vi "controller.vi"() -> ()   [LabVIEW 2017]
uses:
  <vilib>/Instr/_visa.llb/VISA Configure Serial Port (Instr).vi
panel:
  in  "7":bool
  in  "9":bool
  in  "8":bool
  in  "5":bool
  in  "6":bool
  in  "4":bool
  in  "3":bool
  in  "2":bool
  in  "1":bool
  in  "5-3":bool
  in  "5-1":bool
  in  "10-3":bool
  in  "10-2":bool
  in  "10-1":bool
  in  "9-5":bool
  in  "9-4":bool
  in  "9-3":bool
  in  "9-2":bool
  in  "9-1":bool
  in  "8-5":bool
  in  "8-4":bool
  in  "8-3":bool
  in  "8-2":bool
  in  "8-1":bool
  in  "7-5":bool
  in  "7-4":bool
  in  "7-3":bool
  in  "7-2":bool
  in  "7-1":bool
  in  "6-5":bool
  in  "6-4":bool
  in  "6-3":bool
  in  "6-2":bool
  in  "6-1":bool
  in  "5-5":bool
  in  "5-4":bool
  in  "5-2":bool
  in  "4-5":bool
  in  "4-4":bool
  in  "4-3":bool
  in  "4-2":bool
  in  "4-1":bool
  in  "3-5":bool
  in  "3-4":bool
  in  "3-3":bool
  in  "3-2":bool
  in  "3-1":bool
  in  "2-5":bool
  in  "2-4":bool
  in  "2-3":bool
  in  "2-2":bool
  in  "2-1":bool
  in  "1-5":bool
  in  "1-4":bool
  in  "1-3":bool
  in  "1-2":bool
  in  "1-1":bool
  in  "关":u16(ring) items=["1", "2", "3", "4", "5", "6", "7", "8", "9", "10", "11", "12", "13", "14", "15", "16", "17", "18", "19", "20", "21", "22", "23", "24", "25", "26", "27", "28", "29", "30", "31", "32", "33", "34", "35", "36", "37", "38", "39", "40", "41", "42", "43", "44", "45", "46", "47", "48"]
  in  "开":u16(ring) items=["1", "2", "3", "4", "5", "6", "7", "8", "9", "10", "11", "12", "13", "14", "15", "16", "17", "18", "19", "20", "21", "22", "23", "24", "25", "26", "27", "28", "29", "30", "31", "32", "33", "34", "35", "36", "37", "38", "39", "40", "41", "42", "43", "44", "45", "46", "47", "48"]
  in  "全关":bool
  in  "全开":bool
  in  "控制板":refnum<visa-resource-name>="COM9"
  in  "退出":bool
  in  "传感器预热完成":bool
  in  "传感器预热":bool
  in  "流程测试":bool
  in  "测试":bool
  in  "传感器数目":i32=9
  # "控制板调试"
  # "注意：\n因串口带宽、通信时延与寄存器读写操作，\n点击按钮后请等待反应。不要反复点击。"
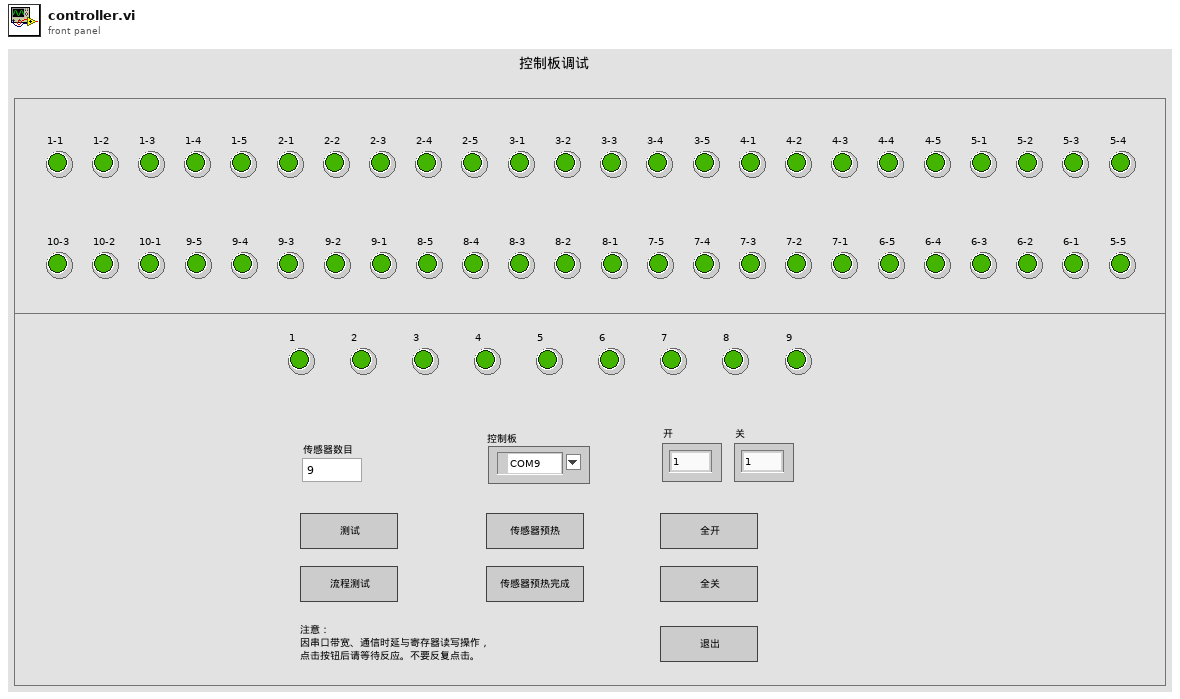
[diagram p1: front panel]
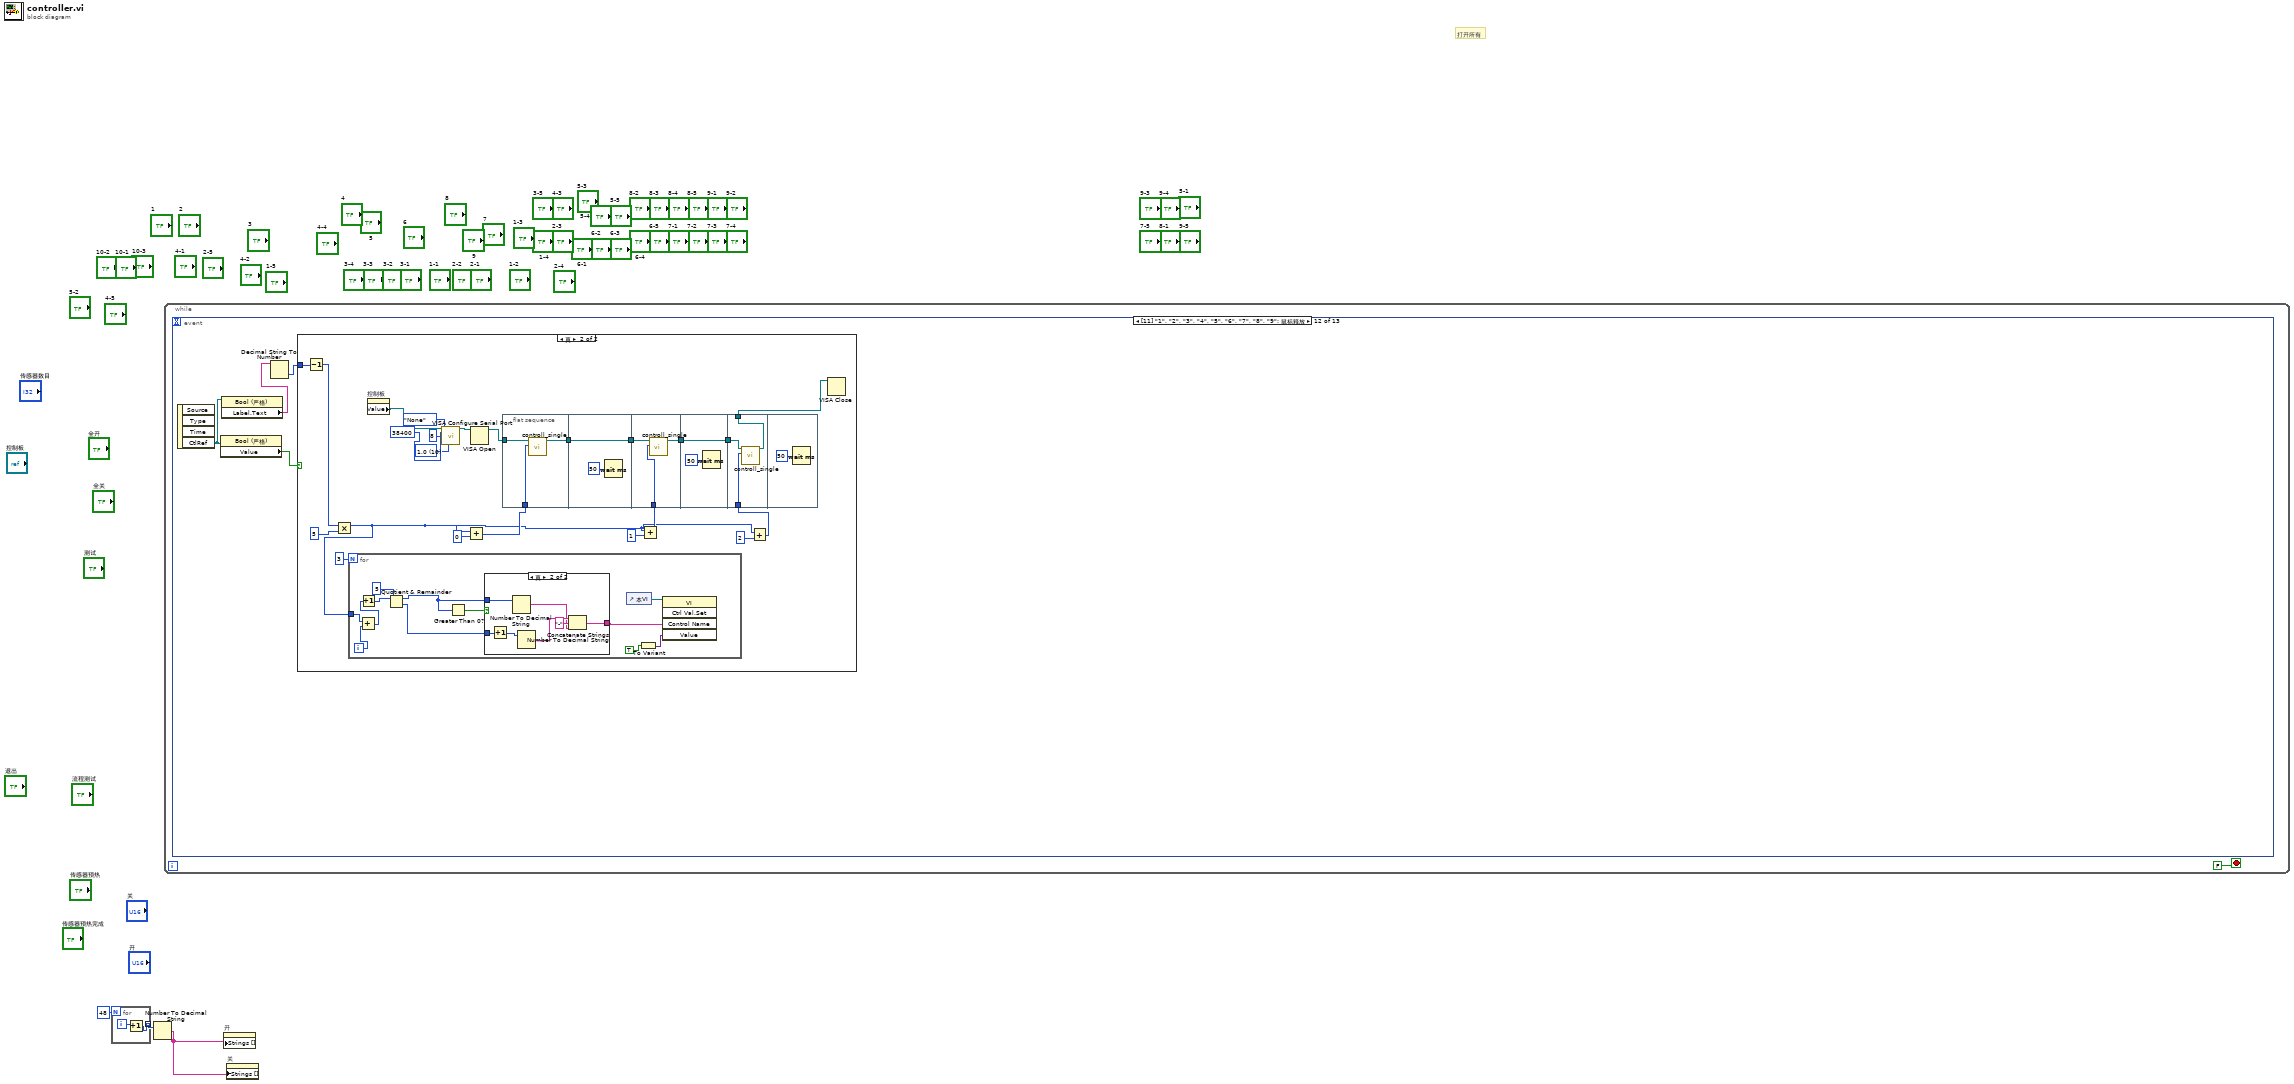
[diagram p0: block diagram]
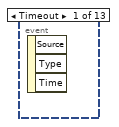
[diagram p2: hidden frame]
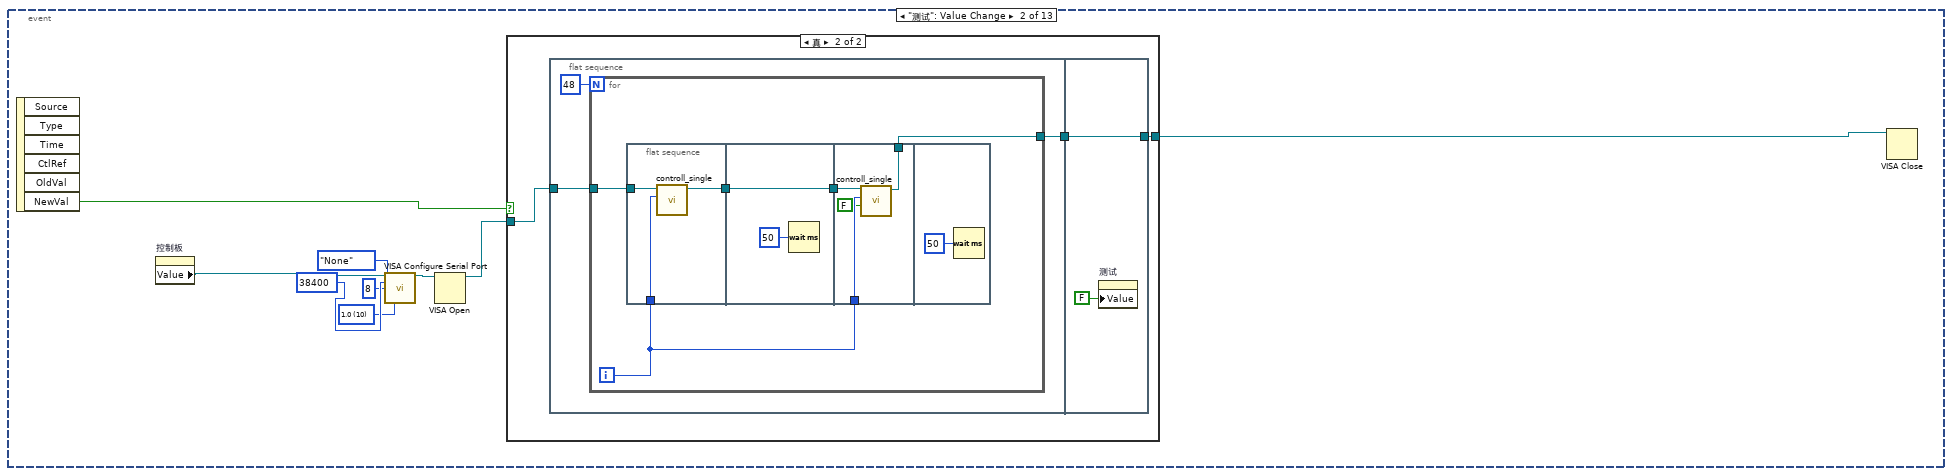
[diagram p3: hidden frame]
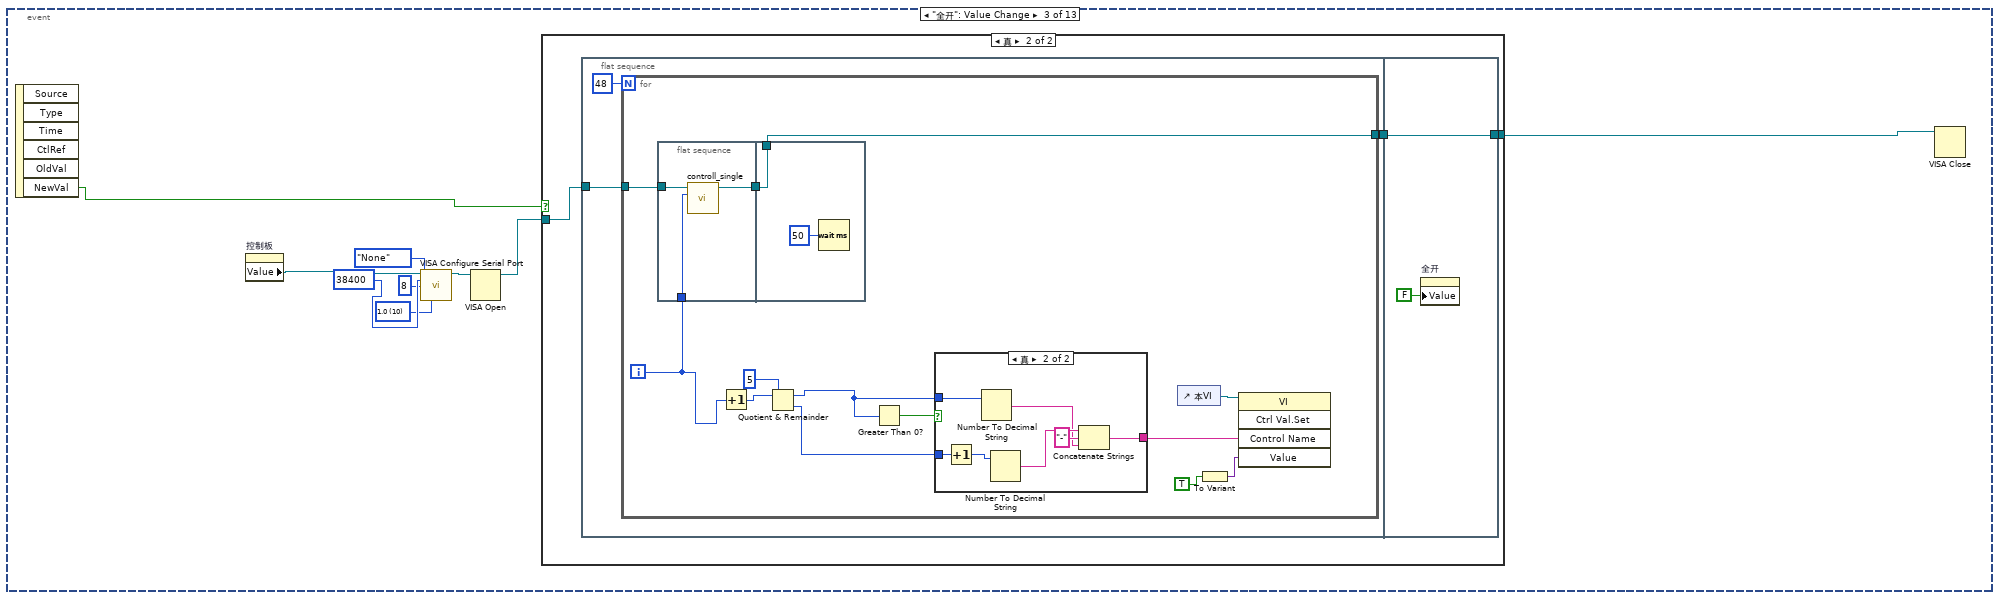
[diagram p5: hidden frame]
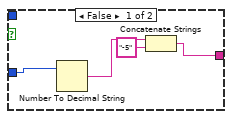
[diagram p7: hidden frame]
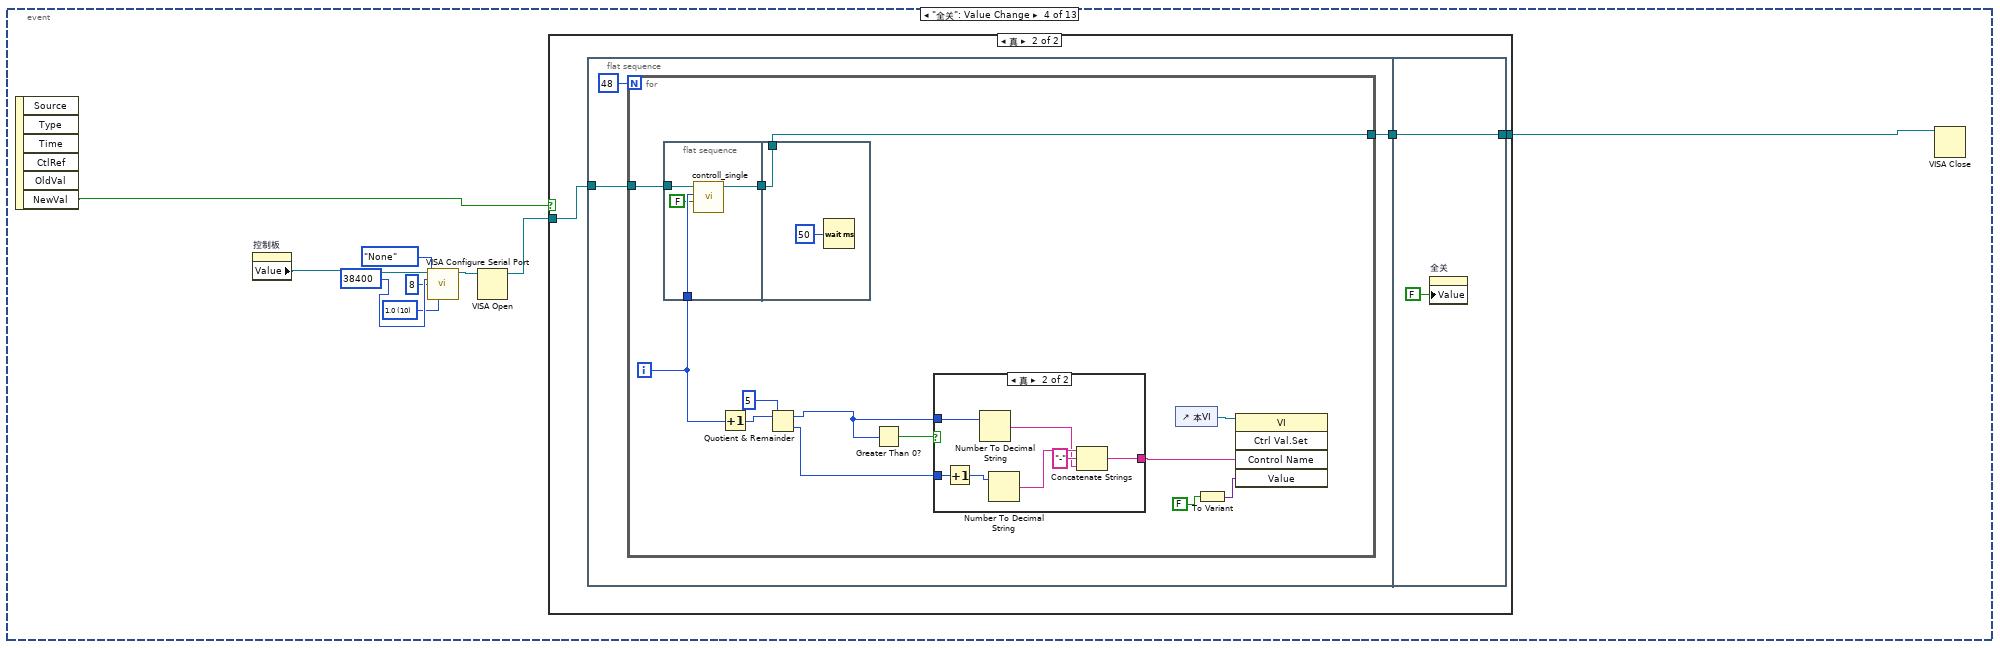
[diagram p8: hidden frame]
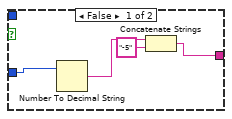
[diagram p10: hidden frame]
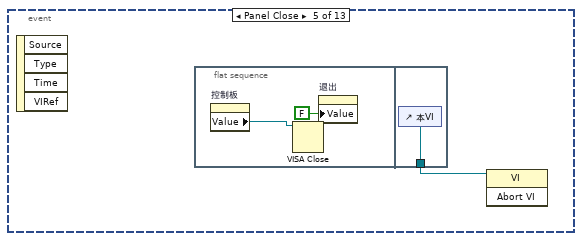
[diagram p11: hidden frame]
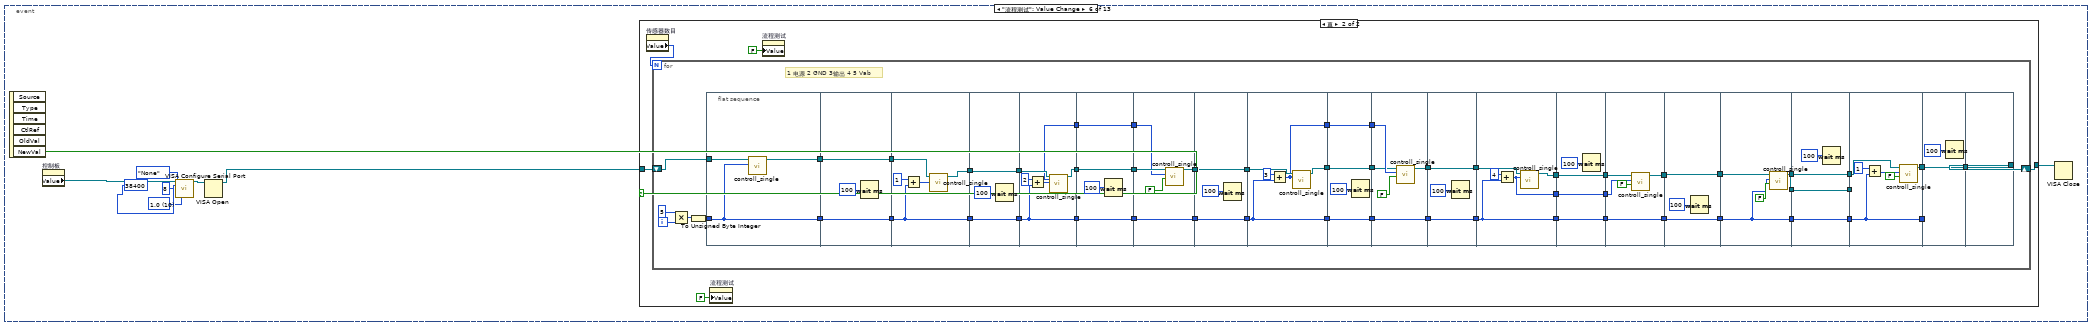
[diagram p12: hidden frame]
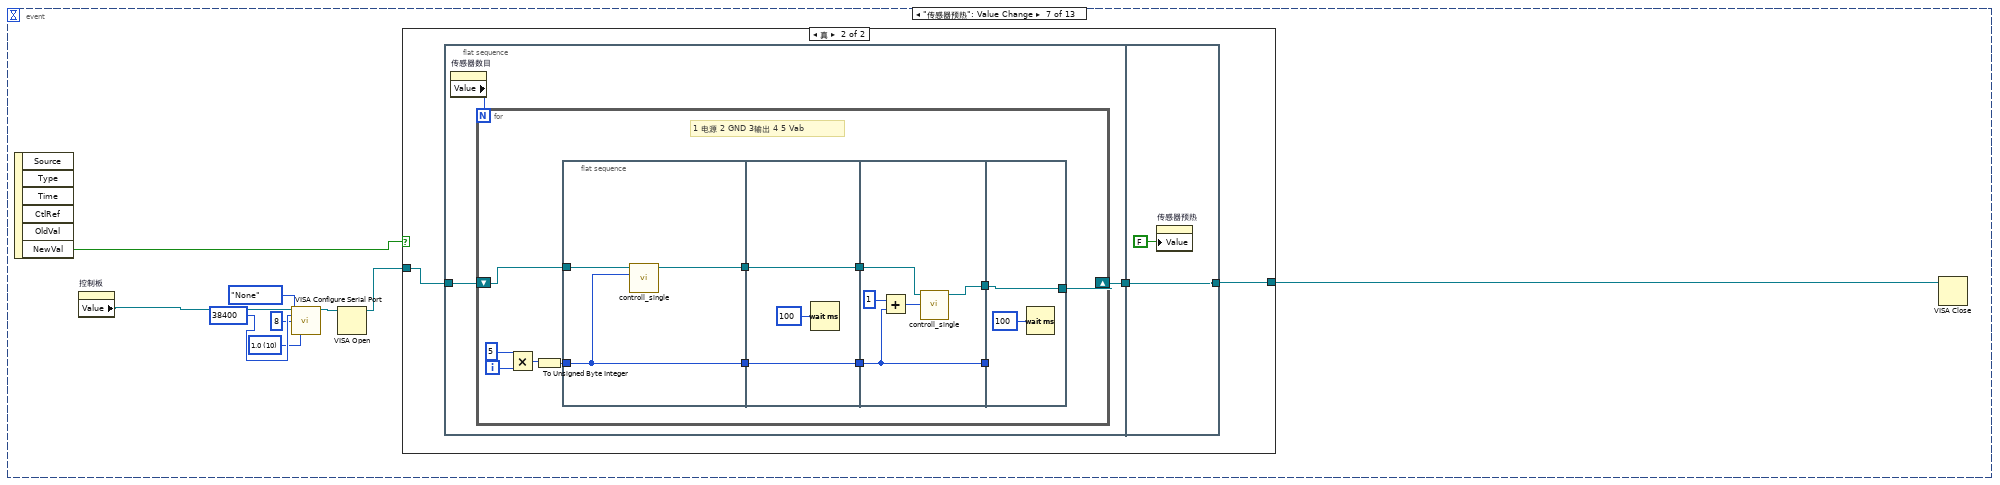
[diagram p14: hidden frame]
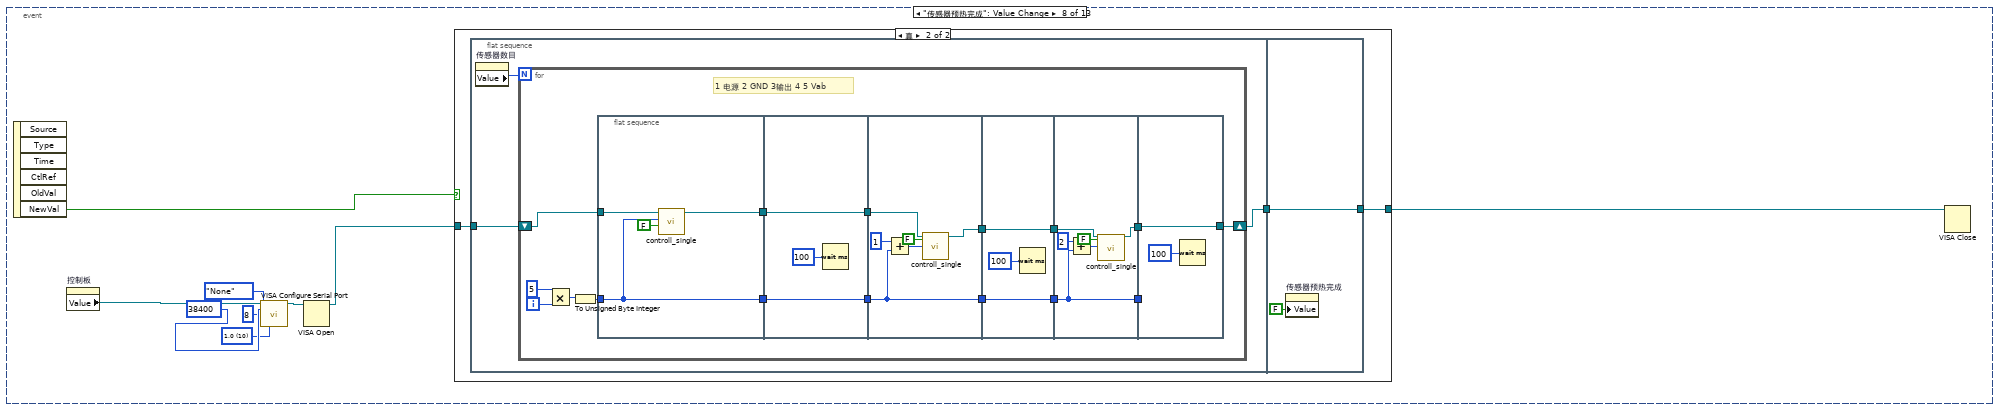
[diagram p16: hidden frame]
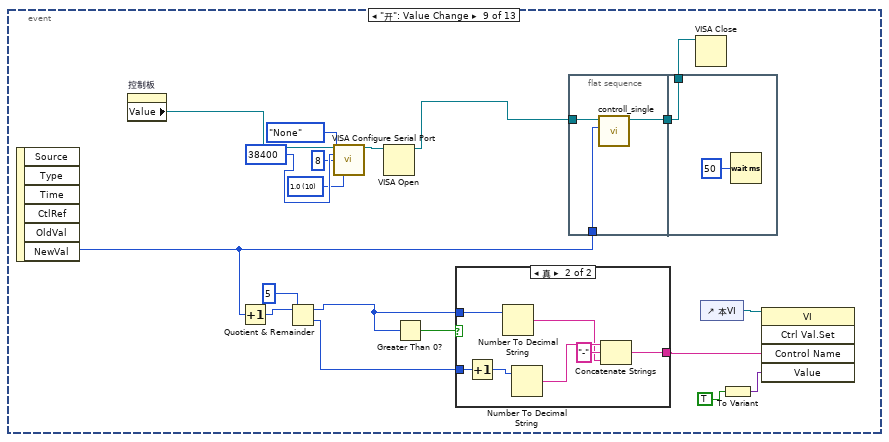
[diagram p18: hidden frame]
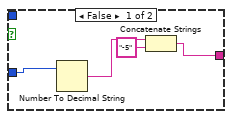
[diagram p19: hidden frame]
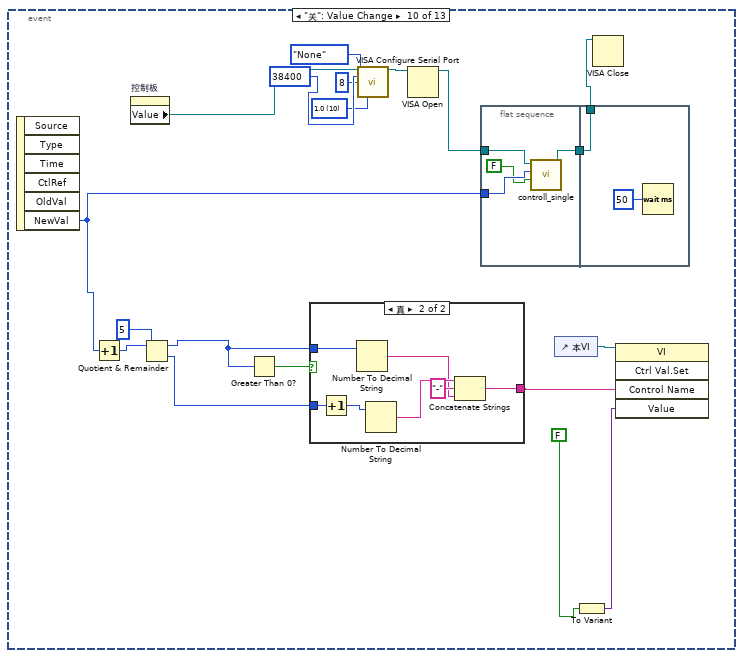
[diagram p20: hidden frame]
diagram:
  # "打开所有"
  n1 = for {
    N: 48 -> [_]
    tunnel: [w4] -> w2 mode=indexing
    i -> [w5]
    n2 = Increment(x=w5) -> (x+1=w4:i32)
  }
  n3 = Number To Decimal String(number=w2) -> (decimal integer string=w1:string[])  [unwired: 1 in]
  n4 = while {
    stop <- FALSE stop-if-true
    n5 = event shown="[11] \"1\", \"2\", \"3\", \"4\", \"5\", \"6\", \"7\", \"8\", \"9\": 鼠标释放" {
      selector: _ -> [_ _ _ _ _ _ _ _ _ _ _ _ _]
      dyn-events: _ -> [_ _ _ _ _ _ _ _ _ _ _ _ _]
      timeout: _ -> [_ _ _ _ _ _ _ _ _ _ _ _ _]
      event Timeout {
        n6 = event-data() -> ()  [unwired: 1 in, 3 out]
      }
      event "测试": Value Change {
        w10 = u16 10 items=["1.0"=10, "1.5"=15, "2.0"=20] ("stop bits (10: 1 bit)")
        n7 = event-data() -> ("NewVal"=w15:bool)  [unwired: 1 in, 5 out]
        n8 = property on="控制板" class="VISAName"() -> ("Value"=w8:refnum<visa-resource-name>)  [unwired: 2 in, 2 out]
        n9 = call-poly "VISA Configure Serial Port"("VISA resource name"=w8, "baud rate (9600)"=u32 38400, "data bits (8)"=u16 8, "parity (0:none)"=enum16{"None", "Odd", "Even", "Mark", "Space"}."None", "stop bits (10: 1 bit)"=w10) -> ("VISA resource name out"=w14:refnum<visa-resource-name>)  [unwired: 9 in, 1 out]
        n10 = VISA Open(VISA resource name=w14) -> (VISA resource name=w9:refnum<visa-resource-name>)  [unwired: 4 in, 1 out]
        n11 = case shown="真" w15 {
          tunnel: w9 -> [w16 w19]
          tunnel: [w16 w18] -> w7
          frame False {
          }
          frame True {
            n12 = flat-sequence {
              tunnel: w19 -> [w21]
              tunnel: [w20] -> w17
              tunnel: [w39] -> w18
              tunnel: w17 -> [w39]
              frame #0 {
                n13 = for {
                  N: 48 -> [_]
                  tunnel: w21 -> [w24]
                  tunnel: [w23] -> w20
                  i -> [w25]
                  n14 = flat-sequence {
                    tunnel: [w30] -> w26
                    tunnel: w25 -> [w29]
                    tunnel: w24 -> [w28]
                    tunnel: [w31] -> w27
                    tunnel: w26 -> [w31]
                    tunnel: w27 -> [w36]
                    tunnel: w25 -> [w35]
                    tunnel: [w33] -> w23
                    frame #0 {
                      n15 = call "controll_single.vi"("控制编号"=w29, "VISA资源名称"=w28) -> ("VISA资源名称输出"=w30:refnum<visa-resource-name>)  [unwired: 9 in]
                    }
                    frame #1 {
                      n16 = Wait (ms)(milliseconds to wait=u32 50 ("等待时间（毫秒）")) -> ()  [unwired: 1 out]
                    }
                    frame #2 {
                      n17 = call "controll_single.vi"("开关"=FALSE, "控制编号"=w35, "VISA资源名称"=w36) -> ("VISA资源名称输出"=w33:refnum<visa-resource-name>)  [unwired: 8 in]
                    }
                    frame #3 {
                      n18 = Wait (ms)(milliseconds to wait=u32 50 ("等待时间（毫秒）")) -> ()  [unwired: 1 out]
                    }
                  }
                }
              }
              frame #1 {
                n19 = property on="测试" class="Bool (严格)"("Value"=FALSE ("测试")) -> ()  [unwired: 2 in, 2 out]
              }
            }
          }
        }
        n20 = VISA Close(VISA resource name=w7) -> ()  [unwired: 1 in, 1 out]
      }
      event "全开": Value Change {
        w44 = u16 10 items=["1.0"=10, "1.5"=15, "2.0"=20] ("stop bits (10: 1 bit)")
        n21 = event-data() -> ("NewVal"=w40:bool)  [unwired: 1 in, 5 out]
        n22 = property on="控制板" class="VISAName"() -> ("Value"=w42:refnum<visa-resource-name>)  [unwired: 2 in, 2 out]
        n23 = call-poly "VISA Configure Serial Port"("VISA resource name"=w42, "baud rate (9600)"=u32 38400, "data bits (8)"=u16 8, "parity (0:none)"=enum16{"None", "Odd", "Even", "Mark", "Space"}."None", "stop bits (10: 1 bit)"=w44) -> ("VISA resource name out"=w48:refnum<visa-resource-name>)  [unwired: 9 in, 1 out]
        n24 = VISA Open(VISA resource name=w48) -> (VISA resource name=w43:refnum<visa-resource-name>)  [unwired: 4 in, 1 out]
        n25 = case shown="真" w40 {
          tunnel: w43 -> [w49 w52]
          tunnel: [w49 w51] -> w41
          frame False {
          }
          frame True {
            n26 = flat-sequence {
              tunnel: w52 -> [w54]
              tunnel: [w53] -> w50
              tunnel: [w86] -> w51
              tunnel: w50 -> [w86]
              frame #0 {
                n27 = for {
                  N: 48 -> [_]
                  tunnel: w54 -> [w67]
                  tunnel: [w66] -> w53
                  i -> [w65]
                  n28 = flat-sequence {
                    tunnel: [w82] -> w68
                    tunnel: w65 -> [w81]
                    tunnel: w67 -> [w80]
                    tunnel: w68 -> [w83]
                    tunnel: [w83] -> w66
                    frame #0 {
                      n29 = call "controll_single.vi"("控制编号"=w81, "VISA资源名称"=w80) -> ("VISA资源名称输出"=w82:refnum<visa-resource-name>)  [unwired: 9 in]
                    }
                    frame #1 {
                      n30 = Wait (ms)(milliseconds to wait=u32 50 ("等待时间（毫秒）")) -> ()  [unwired: 1 out]
                    }
                  }
                  n31 = Increment(x=w65) -> (x+1=w64:i32)
                  n32 = Quotient & Remainder(x=w64, y=u16 5) -> (x-y*floor(x/y)=w60:i32, floor(x/y)=w61:i32)
                  n33 = Greater Than 0?(x=w60) -> (x > 0?=w62:bool)
                  n34 = case shown="真" w62 {
                    tunnel: w61 -> [w70 w79]
                    tunnel: w60 -> [_ w77]
                    tunnel: [w69 w73] -> w58
                    frame False {
                      n35 = Number To Decimal String(number=w70) -> (decimal integer string=w72:string)  [unwired: 1 in]
                      n36 = Concatenate Strings(w72, "-5" ("字符串")) -> (w69:string)
                    }
                    frame True {
                      n37 = Increment(x=w79) -> (x+1=w78:i32)
                      n38 = Number To Decimal String(number=w77) -> (decimal integer string=w74:string)  [unwired: 1 in]
                      n39 = Number To Decimal String(number=w78) -> (decimal integer string=w76:string)  [unwired: 1 in]
                      n40 = Concatenate Strings(w76, "-" ("字符串"), w74) -> (w73:string)
                    }
                  }
                  n41 = control-ref of="本VI"() -> (w59:refnum<vi>)
                  n42 = To Variant(anything=TRUE) -> (Variant=w56:variant)
                  n43 = invoke class="VI" method="Ctrl Val.Set"(reference=w59, "Control Name"=w58, "Value"=w56) -> ()  [unwired: 2 in, 5 out]
                }
              }
              frame #1 {
                n44 = property on="全开" class="Bool (严格)"("Value"=FALSE ("测试")) -> ()  [unwired: 2 in, 2 out]
              }
            }
          }
        }
        n45 = VISA Close(VISA resource name=w41) -> ()  [unwired: 1 in, 1 out]
      }
      event "全关": Value Change {
        w91 = u16 10 items=["1.0"=10, "1.5"=15, "2.0"=20] ("stop bits (10: 1 bit)")
        n46 = event-data() -> ("NewVal"=w87:bool)  [unwired: 1 in, 5 out]
        n47 = property on="控制板" class="VISAName"() -> ("Value"=w89:refnum<visa-resource-name>)  [unwired: 2 in, 2 out]
        n48 = call-poly "VISA Configure Serial Port"("VISA resource name"=w89, "baud rate (9600)"=u32 38400, "data bits (8)"=u16 8, "parity (0:none)"=enum16{"None", "Odd", "Even", "Mark", "Space"}."None", "stop bits (10: 1 bit)"=w91) -> ("VISA resource name out"=w95:refnum<visa-resource-name>)  [unwired: 9 in, 1 out]
        n49 = VISA Open(VISA resource name=w95) -> (VISA resource name=w90:refnum<visa-resource-name>)  [unwired: 4 in, 1 out]
        n50 = case shown="真" w87 {
          tunnel: w90 -> [w96 w99]
          tunnel: [w96 w98] -> w88
          frame False {
          }
          frame True {
            n51 = flat-sequence {
              tunnel: w99 -> [w101]
              tunnel: [w100] -> w97
              tunnel: [w134] -> w98
              tunnel: w97 -> [w134]
              frame #0 {
                n52 = for {
                  N: 48 -> [_]
                  tunnel: w101 -> [w114]
                  tunnel: [w113] -> w100
                  i -> [w103]
                  n53 = flat-sequence {
                    tunnel: [w130] -> w115
                    tunnel: w103 -> [w129]
                    tunnel: w114 -> [w128]
                    tunnel: w115 -> [w131]
                    tunnel: [w131] -> w113
                    frame #0 {
                      n54 = call "controll_single.vi"("开关"=FALSE, "控制编号"=w129, "VISA资源名称"=w128) -> ("VISA资源名称输出"=w130:refnum<visa-resource-name>)  [unwired: 8 in]
                    }
                    frame #1 {
                      n55 = Wait (ms)(milliseconds to wait=u32 50 ("等待时间（毫秒）")) -> ()  [unwired: 1 out]
                    }
                  }
                  n56 = Increment(x=w103) -> (x+1=w112:i32)
                  n57 = Quotient & Remainder(x=w112, y=u16 5) -> (x-y*floor(x/y)=w108:i32, floor(x/y)=w109:i32)
                  n58 = Greater Than 0?(x=w108) -> (x > 0?=w110:bool)
                  n59 = case shown="真" w110 {
                    tunnel: w109 -> [w117 w126]
                    tunnel: w108 -> [_ w124]
                    tunnel: [w116 w120] -> w106
                    frame False {
                      n60 = Number To Decimal String(number=w117) -> (decimal integer string=w119:string)  [unwired: 1 in]
                      n61 = Concatenate Strings(w119, "-5" ("字符串")) -> (w116:string)
                    }
                    frame True {
                      n62 = Increment(x=w126) -> (x+1=w125:i32)
                      n63 = Number To Decimal String(number=w124) -> (decimal integer string=w121:string)  [unwired: 1 in]
                      n64 = Number To Decimal String(number=w125) -> (decimal integer string=w123:string)  [unwired: 1 in]
                      n65 = Concatenate Strings(w123, "-" ("字符串"), w121) -> (w120:string)
                    }
                  }
                  n66 = control-ref of="本VI"() -> (w107:refnum<vi>)
                  n67 = To Variant(anything=FALSE) -> (Variant=w104:variant)
                  n68 = invoke class="VI" method="Ctrl Val.Set"(reference=w107, "Control Name"=w106, "Value"=w104) -> ()  [unwired: 2 in, 5 out]
                }
              }
              frame #1 {
                n69 = property on="全关" class="Bool (严格)"("Value"=FALSE ("测试")) -> ()  [unwired: 2 in, 2 out]
              }
            }
          }
        }
        n70 = VISA Close(VISA resource name=w88) -> ()  [unwired: 1 in, 1 out]
      }
      event Panel Close {
        n71 = event-data() -> ()  [unwired: 1 in, 4 out]
        n72 = flat-sequence {
          tunnel: [w138] -> w135
          frame #0 {
            n73 = property on="控制板" class="VISAName"() -> ("Value"=w136:refnum<visa-resource-name>)  [unwired: 2 in, 2 out]
            n74 = VISA Close(VISA resource name=w136) -> ()  [unwired: 1 in, 1 out]
            n75 = property on="退出" class="Bool (严格)"("Value"=FALSE ("退出")) -> ()  [unwired: 2 in, 2 out]
          }
          frame #1 {
            n76 = control-ref of="本VI"() -> (w138:refnum<vi>)
          }
        }
        n77 = invoke class="VI" method="Abort VI"(reference=w135) -> ()  [unwired: 2 in, 3 out]
      }
      event "流程测试": Value Change {
        w142 = u16 10 items=["1.0"=10, "1.5"=15, "2.0"=20] ("stop bits (10: 1 bit)")
        n78 = event-data() -> ("NewVal"=w147:bool)  [unwired: 1 in, 5 out]
        n79 = property on="控制板" class="VISAName"() -> ("Value"=w141:refnum<visa-resource-name>)  [unwired: 2 in, 2 out]
        n80 = call-poly "VISA Configure Serial Port"("VISA resource name"=w141, "baud rate (9600)"=u32 38400, "data bits (8)"=u16 8, "parity (0:none)"=enum16{"None", "Odd", "Even", "Mark", "Space"}."None", "stop bits (10: 1 bit)"=w142) -> ("VISA resource name out"=w146:refnum<visa-resource-name>)  [unwired: 9 in, 1 out]
        n81 = VISA Open(VISA resource name=w146) -> (VISA resource name=w140:refnum<visa-resource-name>)  [unwired: 4 in, 1 out]
        n82 = case shown="真" w147 {
          tunnel: w140 -> [w148 w153]
          tunnel: [w148 w152] -> w139
          frame False {
          }
          frame True {
            n83 = property on="传感器数目" class="DigNum (严格)"() -> ("Value"=w151:i32)  [unwired: 2 in, 2 out]
            n84 = for {
              N: w151 -> [_]
              shift-right: [w160] -> w152
              shift-left: w153 -> [w202]
              i -> [w206]
              # "1 电源 2 GND 3输出 4 5 Vab"
              n85 = Multiply(x=5, y=w206) -> (x*y=w204:i32)
              n86 = To Unsigned Byte Integer(number=w204) -> (unsigned 8bit integer=w203:u8)
              n87 = flat-sequence {
                tunnel: w202 -> [w209]
                tunnel: [w208] -> w201
                tunnel: w203 -> [w207]
                tunnel: [w207] -> w199
                tunnel: w201 -> [w212]
                tunnel: [w212] -> w200
                tunnel: w199 -> [w211]
                tunnel: [w211] -> w198
                tunnel: w200 -> [w214]
                tunnel: w198 -> [w216]
                tunnel: [w216] -> w197
                tunnel: [w213] -> w195
                tunnel: w197 -> [w220]
                tunnel: [w220] -> w196
                tunnel: w195 -> [w219]
                tunnel: [w219] -> w194
                tunnel: w196 -> [w224]
                tunnel: [w224] -> w193
                tunnel: w194 -> [w223]
                tunnel: [w222] -> w191
                tunnel: [w221] -> w189
                tunnel: w193 -> [w229]
                tunnel: [w229] -> w192
                tunnel: w191 -> [w228]
                tunnel: [w228] -> w190
                tunnel: w189 -> [w227]
                tunnel: [w227] -> w188
                tunnel: w192 -> [w234]
                tunnel: [w234] -> w178
                tunnel: w190 -> [w233]
                tunnel: w188 -> [w232]
                tunnel: [w230] -> w176
                tunnel: w178 -> [w237]
                tunnel: [w237] -> w177
                tunnel: w176 -> [w236]
                tunnel: [w236] -> w175
                tunnel: w177 -> [w241]
                tunnel: [w241] -> w181
                tunnel: [w239] -> w180
                tunnel: [w238] -> w179
                tunnel: w175 -> [w242]
                tunnel: w181 -> [w246]
                tunnel: [w246] -> w187
                tunnel: w180 -> [w245]
                tunnel: [w245] -> w186
                tunnel: w179 -> [w244]
                tunnel: [w244] -> w185
                tunnel: w187 -> [w251]
                tunnel: [w251] -> w171
                tunnel: w186 -> [w248]
                tunnel: w185 -> [w250]
                tunnel: [w247] -> w169
                tunnel: w171 -> [w254]
                tunnel: [w254] -> w170
                tunnel: w169 -> [w253]
                tunnel: [w253] -> w168
                tunnel: w170 -> [w258]
                tunnel: [w258] -> w174
                tunnel: [w255] -> w173
                tunnel: [w256] -> w172
                tunnel: w168 -> [w259]
                tunnel: w174 -> [w263]
                tunnel: [w263] -> w184
                tunnel: w173 -> [w262]
                tunnel: [w262] -> w183
                tunnel: w172 -> [w261]
                tunnel: [w261] -> w182
                tunnel: w184 -> [w265]
                tunnel: w183 -> [w268]
                tunnel: w182 -> [w266]
                tunnel: [w265] -> w167
                tunnel: [w264] -> w165
                tunnel: w167 -> [w271]
                tunnel: [w271] -> w166
                tunnel: w165 -> [w270]
                tunnel: [w270] -> w164
                tunnel: [w272] -> w159
                tunnel: w166 -> [w274]
                tunnel: w164 -> [w273]
                tunnel: [w274] -> w157
                tunnel: [w272] -> w155
                tunnel: w159 -> [w279]
                tunnel: [w279] -> w158
                tunnel: w157 -> [w278]
                tunnel: [w278] -> w156
                tunnel: w155 -> [w277]
                tunnel: [w277] -> w154
                tunnel: w158 -> [_]
                tunnel: [w282] -> w163
                tunnel: w156 -> [w282]
                tunnel: w154 -> [w281]
                tunnel: [w280] -> w161
                tunnel: w163 -> [_]
                tunnel: [w287] -> w162
                tunnel: w161 -> [w287]
                tunnel: w162 -> [w288]
                tunnel: [w288] -> w160
                frame #0 {
                  n88 = call "controll_single.vi"("控制编号"=w207, "VISA资源名称"=w209) -> ("VISA资源名称输出"=w208:refnum<visa-resource-name>)  [unwired: 9 in]
                }
                frame #1 {
                  n89 = Wait (ms)(milliseconds to wait=u32 100 ("等待时间（毫秒）")) -> ()  [unwired: 1 out]
                }
                frame #2 {
                  n90 = Add(x=u8 1, y=w216) -> (x+y=w215:u8)
                  n91 = call "controll_single.vi"("控制编号"=w215, "VISA资源名称"=w214) -> ("VISA资源名称输出"=w213:refnum<visa-resource-name>)  [unwired: 9 in]
                }
                frame #3 {
                  n92 = Wait (ms)(milliseconds to wait=u32 100 ("等待时间（毫秒）")) -> ()  [unwired: 1 out]
                }
                frame #4 {
                  n93 = Add(x=u8 2, y=w224) -> (x+y=w221:u8)
                  n94 = call "controll_single.vi"("控制编号"=w221, "VISA资源名称"=w223) -> ("VISA资源名称输出"=w222:refnum<visa-resource-name>)  [unwired: 9 in]
                }
                frame #5 {
                  n95 = Wait (ms)(milliseconds to wait=u32 100 ("等待时间（毫秒）")) -> ()  [unwired: 1 out]
                }
                frame #6 {
                  n96 = call "controll_single.vi"("开关"=FALSE, "控制编号"=w232, "VISA资源名称"=w233) -> ("VISA资源名称输出"=w230:refnum<visa-resource-name>)  [unwired: 8 in]
                }
                frame #7 {
                  n97 = Wait (ms)(milliseconds to wait=u32 100 ("等待时间（毫秒）")) -> ()  [unwired: 1 out]
                }
                frame #8 {
                  n98 = Add(x=u8 3, y=w241) -> (x+y=w238:u8)
                  n99 = call "controll_single.vi"("控制编号"=w238, "VISA资源名称"=w242) -> ("VISA资源名称输出"=w239:refnum<visa-resource-name>)  [unwired: 9 in]
                }
                frame #9 {
                  n100 = Wait (ms)(milliseconds to wait=u32 100 ("等待时间（毫秒）")) -> ()  [unwired: 1 out]
                }
                frame #10 {
                  n101 = call "controll_single.vi"("开关"=FALSE, "控制编号"=w250, "VISA资源名称"=w248) -> ("VISA资源名称输出"=w247:refnum<visa-resource-name>)  [unwired: 8 in]
                }
                frame #11 {
                  n102 = Wait (ms)(milliseconds to wait=u32 100 ("等待时间（毫秒）")) -> ()  [unwired: 1 out]
                }
                frame #12 {
                  n103 = Add(x=u8 4, y=w258) -> (x+y=w255:u8)
                  n104 = call "controll_single.vi"("控制编号"=w255, "VISA资源名称"=w259) -> ("VISA资源名称输出"=w256:refnum<visa-resource-name>)  [unwired: 9 in]
                }
                frame #13 {
                  n105 = Wait (ms)(milliseconds to wait=u32 100 ("等待时间（毫秒）")) -> ()  [unwired: 1 out]
                }
                frame #14 {
                  n106 = call "controll_single.vi"("开关"=FALSE, "控制编号"=w268, "VISA资源名称"=w266) -> ("VISA资源名称输出"=w264:refnum<visa-resource-name>)  [unwired: 8 in]
                }
                frame #15 {
                  n107 = Wait (ms)(milliseconds to wait=u32 100 ("等待时间（毫秒）")) -> ()  [unwired: 1 out]
                }
                frame #16 {
                  n108 = call "controll_single.vi"("开关"=FALSE, "控制编号"=w274, "VISA资源名称"=w273) -> ("VISA资源名称输出"=w272:refnum<visa-resource-name>)  [unwired: 8 in]
                }
                frame #17 {
                  n109 = Wait (ms)(milliseconds to wait=u32 100 ("等待时间（毫秒）")) -> ()  [unwired: 1 out]
                }
                frame #18 {
                  n110 = Add(x=u8 1, y=w282) -> (x+y=w285:u8)
                  n111 = call "controll_single.vi"("开关"=FALSE, "控制编号"=w285, "VISA资源名称"=w281) -> ("VISA资源名称输出"=w280:refnum<visa-resource-name>)  [unwired: 8 in]
                }
                frame #19 {
                  n112 = Wait (ms)(milliseconds to wait=u32 100 ("等待时间（毫秒）")) -> ()  [unwired: 1 out]
                }
                frame #20 {
                }
              }
            }
            n113 = property on="流程测试" class="Bool (严格)"("Value"=FALSE ("流程测试")) -> ()  [unwired: 2 in, 2 out]
            n114 = property on="流程测试" class="Bool (严格)"("Value"=FALSE ("流程测试")) -> ()  [unwired: 2 in, 2 out]
          }
        }
        n115 = VISA Close(VISA resource name=w139) -> ()  [unwired: 1 in, 1 out]
      }
      event "传感器预热": Value Change {
        w292 = u16 10 items=["1.0"=10, "1.5"=15, "2.0"=20] ("stop bits (10: 1 bit)")
        n116 = event-data() -> ("NewVal"=w297:bool)  [unwired: 1 in, 5 out]
        n117 = property on="控制板" class="VISAName"() -> ("Value"=w291:refnum<visa-resource-name>)  [unwired: 2 in, 2 out]
        n118 = call-poly "VISA Configure Serial Port"("VISA resource name"=w291, "baud rate (9600)"=u32 38400, "data bits (8)"=u16 8, "parity (0:none)"=enum16{"None", "Odd", "Even", "Mark", "Space"}."None", "stop bits (10: 1 bit)"=w292) -> ("VISA resource name out"=w296:refnum<visa-resource-name>)  [unwired: 9 in, 1 out]
        n119 = VISA Open(VISA resource name=w296) -> (VISA resource name=w290:refnum<visa-resource-name>)  [unwired: 4 in, 1 out]
        n120 = case shown="真" w297 {
          tunnel: [w298 w301] -> w289
          tunnel: w290 -> [w298 w300]
          frame False {
          }
          frame True {
            n121 = flat-sequence {
              tunnel: w300 -> [w302]
              tunnel: [w303] -> w299
              tunnel: [w331] -> w301
              tunnel: w299 -> [w331]
              frame #0 {
                n122 = property on="传感器数目" class="DigNum (严格)"() -> ("Value"=w304:i32)  [unwired: 2 in, 2 out]
                n123 = for {
                  N: w304 -> [_]
                  shift-right: [w305] -> w303
                  shift-left: w302 -> [w312]
                  i -> [w316]
                  # "1 电源 2 GND 3输出 4 5 Vab"
                  n124 = Multiply(x=5, y=w316) -> (x*y=w314:i32)
                  n125 = To Unsigned Byte Integer(number=w314) -> (unsigned 8bit integer=w313:u8)
                  n126 = flat-sequence {
                    tunnel: w312 -> [w319]
                    tunnel: [w318] -> w311
                    tunnel: w313 -> [w317]
                    tunnel: [w317] -> w309
                    tunnel: w311 -> [w322]
                    tunnel: [w322] -> w310
                    tunnel: w309 -> [w321]
                    tunnel: [w321] -> w308
                    tunnel: w310 -> [w324]
                    tunnel: w308 -> [w326]
                    tunnel: [w326] -> w307
                    tunnel: [w323] -> w306
                    tunnel: w307 -> [_]
                    tunnel: w306 -> [w328]
                    tunnel: [w328] -> w305
                    frame #0 {
                      n127 = call "controll_single.vi"("控制编号"=w317, "VISA资源名称"=w319) -> ("VISA资源名称输出"=w318:refnum<visa-resource-name>)  [unwired: 9 in]
                    }
                    frame #1 {
                      n128 = Wait (ms)(milliseconds to wait=u32 100 ("等待时间（毫秒）")) -> ()  [unwired: 1 out]
                    }
                    frame #2 {
                      n129 = Add(x=u8 1, y=w326) -> (x+y=w325:u8)
                      n130 = call "controll_single.vi"("控制编号"=w325, "VISA资源名称"=w324) -> ("VISA资源名称输出"=w323:refnum<visa-resource-name>)  [unwired: 9 in]
                    }
                    frame #3 {
                      n131 = Wait (ms)(milliseconds to wait=u32 100 ("等待时间（毫秒）")) -> ()  [unwired: 1 out]
                    }
                  }
                }
              }
              frame #1 {
                n132 = property on="传感器预热" class="Bool (严格)"("Value"=FALSE ("传感器预热")) -> ()  [unwired: 2 in, 2 out]
              }
            }
          }
        }
        n133 = VISA Close(VISA resource name=w289) -> ()  [unwired: 1 in, 1 out]
      }
      event "传感器预热完成": Value Change {
        w335 = u16 10 items=["1.0"=10, "1.5"=15, "2.0"=20] ("stop bits (10: 1 bit)")
        n134 = event-data() -> ("NewVal"=w340:bool)  [unwired: 1 in, 5 out]
        n135 = property on="控制板" class="VISAName"() -> ("Value"=w334:refnum<visa-resource-name>)  [unwired: 2 in, 2 out]
        n136 = call-poly "VISA Configure Serial Port"("VISA resource name"=w334, "baud rate (9600)"=u32 38400, "data bits (8)"=u16 8, "parity (0:none)"=enum16{"None", "Odd", "Even", "Mark", "Space"}."None", "stop bits (10: 1 bit)"=w335) -> ("VISA resource name out"=w339:refnum<visa-resource-name>)  [unwired: 9 in, 1 out]
        n137 = VISA Open(VISA resource name=w339) -> (VISA resource name=w333:refnum<visa-resource-name>)  [unwired: 4 in, 1 out]
        n138 = case shown="真" w340 {
          tunnel: w333 -> [w341 w344]
          tunnel: [w341 w343] -> w332
          frame False {
          }
          frame True {
            n139 = flat-sequence {
              tunnel: w344 -> [w347]
              tunnel: [w345] -> w342
              tunnel: [w389] -> w343
              tunnel: w342 -> [w389]
              frame #0 {
                n140 = property on="传感器数目" class="DigNum (严格)"() -> ("Value"=w346:i32)  [unwired: 2 in, 2 out]
                n141 = for {
                  N: w346 -> [_]
                  shift-right: [w348] -> w345
                  shift-left: w347 -> [w359]
                  i -> [w363]
                  # "1 电源 2 GND 3输出 4 5 Vab"
                  n142 = Multiply(x=5, y=w363) -> (x*y=w361:i32)
                  n143 = To Unsigned Byte Integer(number=w361) -> (unsigned 8bit integer=w360:u8)
                  n144 = flat-sequence {
                    tunnel: w359 -> [w367]
                    tunnel: [w366] -> w358
                    tunnel: w360 -> [w365]
                    tunnel: [w365] -> w356
                    tunnel: w358 -> [w370]
                    tunnel: [w370] -> w357
                    tunnel: w356 -> [w369]
                    tunnel: [w369] -> w355
                    tunnel: w357 -> [w373]
                    tunnel: w355 -> [w375]
                    tunnel: [w375] -> w354
                    tunnel: [w372] -> w352
                    tunnel: w354 -> [w379]
                    tunnel: [w379] -> w353
                    tunnel: w352 -> [w378]
                    tunnel: [w378] -> w351
                    tunnel: w353 -> [w384]
                    tunnel: [w384] -> w350
                    tunnel: w351 -> [w383]
                    tunnel: [w382] -> w349
                    tunnel: w350 -> [_]
                    tunnel: w349 -> [w386]
                    tunnel: [w386] -> w348
                    frame #0 {
                      n145 = call "controll_single.vi"("开关"=FALSE, "控制编号"=w365, "VISA资源名称"=w367) -> ("VISA资源名称输出"=w366:refnum<visa-resource-name>)  [unwired: 8 in]
                    }
                    frame #1 {
                      n146 = Wait (ms)(milliseconds to wait=u32 100 ("等待时间（毫秒）")) -> ()  [unwired: 1 out]
                    }
                    frame #2 {
                      n147 = Add(x=u8 1, y=w375) -> (x+y=w374:u8)
                      n148 = call "controll_single.vi"("开关"=FALSE, "控制编号"=w374, "VISA资源名称"=w373) -> ("VISA资源名称输出"=w372:refnum<visa-resource-name>)  [unwired: 8 in]
                    }
                    frame #3 {
                      n149 = Wait (ms)(milliseconds to wait=u32 100 ("等待时间（毫秒）")) -> ()  [unwired: 1 out]
                    }
                    frame #4 {
                      n150 = Add(x=u8 2, y=w384) -> (x+y=w381:u8)
                      n151 = call "controll_single.vi"("开关"=FALSE, "控制编号"=w381, "VISA资源名称"=w383) -> ("VISA资源名称输出"=w382:refnum<visa-resource-name>)  [unwired: 8 in]
                    }
                    frame #5 {
                      n152 = Wait (ms)(milliseconds to wait=u32 100 ("等待时间（毫秒）")) -> ()  [unwired: 1 out]
                    }
                  }
                }
              }
              frame #1 {
                n153 = property on="传感器预热完成" class="Bool (严格)"("Value"=FALSE ("传感器预热完成")) -> ()  [unwired: 2 in, 2 out]
              }
            }
          }
        }
        n154 = VISA Close(VISA resource name=w332) -> ()  [unwired: 1 in, 1 out]
      }
      event "开": Value Change {
        w394 = u16 10 items=["1.0"=10, "1.5"=15, "2.0"=20] ("stop bits (10: 1 bit)")
        n155 = event-data() -> ("NewVal"=w390:u16)  [unwired: 1 in, 5 out]
        n156 = property on="控制板" class="VISAName"() -> ("Value"=w393:refnum<visa-resource-name>)  [unwired: 2 in, 2 out]
        n157 = Increment(x=w390) -> (x+1=w408:u16)
        n158 = Quotient & Remainder(x=w408, y=u16 5) -> (x-y*floor(x/y)=w404:u16, floor(x/y)=w405:u16)
        n159 = call-poly "VISA Configure Serial Port"("VISA resource name"=w393, "baud rate (9600)"=u32 38400, "data bits (8)"=u16 8, "parity (0:none)"=enum16{"None", "Odd", "Even", "Mark", "Space"}."None", "stop bits (10: 1 bit)"=w394) -> ("VISA resource name out"=w398:refnum<visa-resource-name>)  [unwired: 9 in, 1 out]
        n160 = VISA Open(VISA resource name=w398) -> (VISA resource name=w392:refnum<visa-resource-name>)  [unwired: 4 in, 1 out]
        n161 = Greater Than 0?(x=w404) -> (x > 0?=w406:bool)
        n162 = case shown="真" w406 {
          tunnel: w405 -> [w415 w424]
          tunnel: w404 -> [_ w422]
          tunnel: [w414 w418] -> w402
          frame False {
            n163 = Number To Decimal String(number=w415) -> (decimal integer string=w417:string)  [unwired: 1 in]
            n164 = Concatenate Strings(w417, "-5" ("字符串")) -> (w414:string)
          }
          frame True {
            n165 = Increment(x=w424) -> (x+1=w423:u16)
            n166 = Number To Decimal String(number=w422) -> (decimal integer string=w419:string)  [unwired: 1 in]
            n167 = Number To Decimal String(number=w423) -> (decimal integer string=w421:string)  [unwired: 1 in]
            n168 = Concatenate Strings(w421, "-" ("字符串"), w419) -> (w418:string)
          }
        }
        n169 = flat-sequence {
          tunnel: [w411] -> w399
          tunnel: w392 -> [w410]
          tunnel: w390 -> [w409]
          tunnel: w399 -> [w412]
          tunnel: [w412] -> w391
          frame #0 {
            n170 = call "controll_single.vi"("控制编号"=w409, "VISA资源名称"=w410) -> ("VISA资源名称输出"=w411:refnum<visa-resource-name>)  [unwired: 9 in]
          }
          frame #1 {
            n171 = Wait (ms)(milliseconds to wait=u32 50 ("等待时间（毫秒）")) -> ()  [unwired: 1 out]
          }
        }
        n172 = VISA Close(VISA resource name=w391) -> ()  [unwired: 1 in, 1 out]
        n173 = control-ref of="本VI"() -> (w403:refnum<vi>)
        n174 = To Variant(anything=TRUE) -> (Variant=w400:variant)
        n175 = invoke class="VI" method="Ctrl Val.Set"(reference=w403, "Control Name"=w402, "Value"=w400) -> ()  [unwired: 2 in, 5 out]
      }
      event "关": Value Change {
        w439 = u16 10 items=["1.0"=10, "1.5"=15, "2.0"=20] ("stop bits (10: 1 bit)")
        n176 = event-data() -> ("NewVal"=w425:u16)  [unwired: 1 in, 5 out]
        n177 = Increment(x=w425) -> (x+1=w434:u16)
        n178 = property on="控制板" class="VISAName"() -> ("Value"=w438:refnum<visa-resource-name>)  [unwired: 2 in, 2 out]
        n179 = Quotient & Remainder(x=w434, y=u16 5) -> (x-y*floor(x/y)=w430:u16, floor(x/y)=w431:u16)
        n180 = Greater Than 0?(x=w430) -> (x > 0?=w432:bool)
        n181 = case shown="真" w432 {
          tunnel: w431 -> [w445 w454]
          tunnel: w430 -> [_ w452]
          tunnel: [w444 w448] -> w428
          frame False {
            n182 = Number To Decimal String(number=w445) -> (decimal integer string=w447:string)  [unwired: 1 in]
            n183 = Concatenate Strings(w447, "-5" ("字符串")) -> (w444:string)
          }
          frame True {
            n184 = Increment(x=w454) -> (x+1=w453:u16)
            n185 = Number To Decimal String(number=w452) -> (decimal integer string=w449:string)  [unwired: 1 in]
            n186 = Number To Decimal String(number=w453) -> (decimal integer string=w451:string)  [unwired: 1 in]
            n187 = Concatenate Strings(w451, "-" ("字符串"), w449) -> (w448:string)
          }
        }
        n188 = call-poly "VISA Configure Serial Port"("VISA resource name"=w438, "baud rate (9600)"=u32 38400, "data bits (8)"=u16 8, "parity (0:none)"=enum16{"None", "Odd", "Even", "Mark", "Space"}."None", "stop bits (10: 1 bit)"=w439) -> ("VISA resource name out"=w443:refnum<visa-resource-name>)  [unwired: 9 in, 1 out]
        n189 = VISA Open(VISA resource name=w443) -> (VISA resource name=w436:refnum<visa-resource-name>)  [unwired: 4 in, 1 out]
        n190 = flat-sequence {
          tunnel: [w458] -> w437
          tunnel: w436 -> [w457]
          tunnel: w425 -> [w456]
          tunnel: w437 -> [w459]
          tunnel: [w459] -> w435
          frame #0 {
            n191 = call "controll_single.vi"("开关"=FALSE, "控制编号"=w456, "VISA资源名称"=w457) -> ("VISA资源名称输出"=w458:refnum<visa-resource-name>)  [unwired: 8 in]
          }
          frame #1 {
            n192 = Wait (ms)(milliseconds to wait=u32 50 ("等待时间（毫秒）")) -> ()  [unwired: 1 out]
          }
        }
        n193 = control-ref of="本VI"() -> (w429:refnum<vi>)
        n194 = To Variant(anything=FALSE) -> (Variant=w426:variant)
        n195 = VISA Close(VISA resource name=w435) -> ()  [unwired: 1 in, 1 out]
        n196 = invoke class="VI" method="Ctrl Val.Set"(reference=w429, "Control Name"=w428, "Value"=w426) -> ()  [unwired: 2 in, 5 out]
      }
      event "1-1", "1-2", "1-3", "1-4", "1-5", "2-1", "2-2", "2-3", "2-4", "2-5", "3-1", "3-2", "3-3", "3-4", "3-5", "4-1", "4-2", "4-3", "4-4", "4-5", "5-1", "5-2", "5-3", "5-4", "5-5", "6-1", "6-2", "6-3", "6-4", "6-5", "7-1", "7-2", "7-3", "7-4", "7-5", "8-1", "8-2", "8-3", "8-4", "8-5", "9-1", "9-2", "9-3", "9-4", "9-5": Mouse Up {
        n197 = event-data() -> ("CtlRef"=w462:refnum<vi>)  [unwired: 1 in, 7 out]
        n198 = property class="Bool (严格)"(reference=w462) -> ("Value"=w461:bool)  [unwired: 1 in, 2 out]
        n199 = property class="Bool (严格)"(reference=w462) -> ("Label.Text"=w473:string)  [unwired: 1 in, 2 out]
        n200 = Match Pattern(string=w473, regular expression="-" ("正则表达式")) -> (before substring=w471:string, after substring=w470:string)  [unwired: 1 in, 2 out]
        n201 = Decimal String To Number(string=w471) -> (number=w469:i32)  [unwired: 2 in, 1 out]
        n202 = Decimal String To Number(string=w470) -> (number=w465:i32)  [unwired: 2 in, 1 out]
        n203 = Decrement(x=w469) -> (x-1=w468:i32)
        n204 = Multiply(x=5, y=w468) -> (x*y=w466:i32)
        n205 = Add(x=w466, y=w465) -> (x+y=w464:i32)
        n206 = Decrement(x=w464) -> (x-1=w463:i32)
        n207 = case shown="假" w461 {
          tunnel: w463 -> [w474 w490]
          frame False {
            w478 = u16 10 items=["1.0"=10, "1.5"=15, "2.0"=20] ("stop bits (10: 1 bit)")
            n208 = property on="控制板" class="VISAName"() -> ("Value"=w477:refnum<visa-resource-name>)  [unwired: 2 in, 2 out]
            n209 = call-poly "VISA Configure Serial Port"("VISA resource name"=w477, "baud rate (9600)"=u32 38400, "data bits (8)"=u16 8, "parity (0:none)"=enum16{"None", "Odd", "Even", "Mark", "Space"}."None", "stop bits (10: 1 bit)"=w478) -> ("VISA resource name out"=w482:refnum<visa-resource-name>)  [unwired: 9 in, 1 out]
            n210 = VISA Open(VISA resource name=w482) -> (VISA resource name=w476:refnum<visa-resource-name>)  [unwired: 4 in, 1 out]
            n211 = flat-sequence {
              tunnel: [w487] -> w483
              tunnel: w476 -> [w486]
              tunnel: w474 -> [w485]
              tunnel: w483 -> [w488]
              tunnel: [w488] -> w475
              frame #0 {
                n212 = call "controll_single.vi"("开关"=FALSE, "控制编号"=w485, "VISA资源名称"=w486) -> ("VISA资源名称输出"=w487:refnum<visa-resource-name>)  [unwired: 8 in]
              }
              frame #1 {
                n213 = Wait (ms)(milliseconds to wait=u32 50 ("等待时间（毫秒）")) -> ()  [unwired: 1 out]
              }
            }
            n214 = VISA Close(VISA resource name=w475) -> ()  [unwired: 1 in, 1 out]
          }
          frame True {
            w494 = u16 10 items=["1.0"=10, "1.5"=15, "2.0"=20] ("stop bits (10: 1 bit)")
            n215 = property on="控制板" class="VISAName"() -> ("Value"=w493:refnum<visa-resource-name>)  [unwired: 2 in, 2 out]
            n216 = call-poly "VISA Configure Serial Port"("VISA resource name"=w493, "baud rate (9600)"=u32 38400, "data bits (8)"=u16 8, "parity (0:none)"=enum16{"None", "Odd", "Even", "Mark", "Space"}."None", "stop bits (10: 1 bit)"=w494) -> ("VISA resource name out"=w498:refnum<visa-resource-name>)  [unwired: 9 in, 1 out]
            n217 = VISA Open(VISA resource name=w498) -> (VISA resource name=w492:refnum<visa-resource-name>)  [unwired: 4 in, 1 out]
            n218 = flat-sequence {
              tunnel: [w502] -> w499
              tunnel: w492 -> [w501]
              tunnel: w490 -> [w500]
              tunnel: w499 -> [w503]
              tunnel: [w503] -> w491
              frame #0 {
                n219 = call "controll_single.vi"("控制编号"=w500, "VISA资源名称"=w501) -> ("VISA资源名称输出"=w502:refnum<visa-resource-name>)  [unwired: 9 in]
              }
              frame #1 {
                n220 = Wait (ms)(milliseconds to wait=u32 50 ("等待时间（毫秒）")) -> ()  [unwired: 1 out]
              }
            }
            n221 = VISA Close(VISA resource name=w491) -> ()  [unwired: 1 in, 1 out]
          }
        }
      }
      event "1", "2", "3", "4", "5", "6", "7", "8", "9": Mouse Up {
        n222 = event-data() -> ("CtlRef"=w507:refnum<vi>)  [unwired: 1 in, 3 out]
        n223 = property class="Bool (严格)"(reference=w507) -> ("Value"=w508:bool)  [unwired: 1 in, 2 out]
        n224 = property class="Bool (严格)"(reference=w507) -> ("Label.Text"=w506:string)  [unwired: 1 in, 2 out]
        n225 = Decimal String To Number(string=w506) -> (number=w505:i32)  [unwired: 2 in, 1 out]
        n226 = case shown="真" w508 {
          tunnel: w505 -> [w510 w585]
          frame False {
            w523 = u16 10 items=["1.0"=10, "1.5"=15, "2.0"=20] ("stop bits (10: 1 bit)")
            n227 = Decrement(x=w510) -> (x-1=w520:i32)
            n228 = Multiply(x=w520, y=5) -> (x*y=w509:i32)
            n229 = property on="控制板" class="VISAName"() -> ("Value"=w522:refnum<visa-resource-name>)  [unwired: 2 in, 2 out]
            n230 = for {
              N: 3 -> [_]
              tunnel: w509 -> [w533]
              i -> [w532]
              n231 = Add(x=w533, y=w532) -> (x+y=w534:i32)
              n232 = Increment(x=w534) -> (x+1=w543:i32)
              n233 = Quotient & Remainder(x=w543, y=u16 5) -> (x-y*floor(x/y)=w539:i32, floor(x/y)=w540:i32)
              n234 = Greater Than 0?(x=w539) -> (x > 0?=w541:bool)
              n235 = case shown="真" w541 {
                tunnel: w540 -> [w545 w554]
                tunnel: w539 -> [_ w552]
                tunnel: [w544 w548] -> w537
                frame False {
                  n236 = Number To Decimal String(number=w545) -> (decimal integer string=w547:string)  [unwired: 1 in]
                  n237 = Concatenate Strings(w547, "-5" ("字符串")) -> (w544:string)
                }
                frame True {
                  n238 = Increment(x=w554) -> (x+1=w553:i32)
                  n239 = Number To Decimal String(number=w552) -> (decimal integer string=w549:string)  [unwired: 1 in]
                  n240 = Number To Decimal String(number=w553) -> (decimal integer string=w551:string)  [unwired: 1 in]
                  n241 = Concatenate Strings(w551, "-" ("字符串"), w549) -> (w548:string)
                }
              }
              n242 = control-ref of="本VI"() -> (w538:refnum<vi>)
              n243 = To Variant(anything=FALSE) -> (Variant=w535:variant)
              n244 = invoke class="VI" method="Ctrl Val.Set"(reference=w538, "Control Name"=w537, "Value"=w535) -> ()  [unwired: 2 in, 5 out]
            }
            n245 = call-poly "VISA Configure Serial Port"("VISA resource name"=w522, "baud rate (9600)"=u32 38400, "data bits (8)"=u16 8, "parity (0:none)"=enum16{"None", "Odd", "Even", "Mark", "Space"}."None", "stop bits (10: 1 bit)"=w523) -> ("VISA resource name out"=w527:refnum<visa-resource-name>)  [unwired: 9 in, 1 out]
            n246 = Add(x=w509, y=0) -> (x+y=w514:i32)
            n247 = VISA Open(VISA resource name=w527) -> (VISA resource name=w521:refnum<visa-resource-name>)  [unwired: 4 in, 1 out]
            n248 = flat-sequence {
              tunnel: [w558] -> w531
              tunnel: w514 -> [w557]
              tunnel: w521 -> [w556]
              tunnel: w531 -> [w559]
              tunnel: [w559] -> w530
              tunnel: w530 -> [w564]
              tunnel: [w563] -> w529
              tunnel: w515 -> [w562]
              tunnel: w529 -> [w565]
              tunnel: [w565] -> w528
              tunnel: w516 -> [w570]
              tunnel: w528 -> [w569]
              tunnel: [w567] -> w512
              frame #0 {
                n249 = call "controll_single.vi"("开关"=FALSE, "控制编号"=w557, "VISA资源名称"=w556) -> ("VISA资源名称输出"=w558:refnum<visa-resource-name>)  [unwired: 8 in]
              }
              frame #1 {
                n250 = Wait (ms)(milliseconds to wait=u32 50 ("等待时间（毫秒）")) -> ()  [unwired: 1 out]
              }
              frame #2 {
                n251 = call "controll_single.vi"("开关"=FALSE, "控制编号"=w562, "VISA资源名称"=w564) -> ("VISA资源名称输出"=w563:refnum<visa-resource-name>)  [unwired: 8 in]
              }
              frame #3 {
                n252 = Wait (ms)(milliseconds to wait=u32 50 ("等待时间（毫秒）")) -> ()  [unwired: 1 out]
              }
              frame #4 {
                n253 = call "controll_single.vi"("开关"=FALSE, "控制编号"=w570, "VISA资源名称"=w569) -> ("VISA资源名称输出"=w567:refnum<visa-resource-name>)  [unwired: 8 in]
              }
              frame #5 {
                n254 = Wait (ms)(milliseconds to wait=u32 50 ("等待时间（毫秒）")) -> ()  [unwired: 1 out]
              }
            }
            n255 = Add(x=w509, y=1) -> (x+y=w515:i32)
            n256 = Add(x=w509, y=2) -> (x+y=w516:i32)
            n257 = VISA Close(VISA resource name=w512) -> ()  [unwired: 1 in, 1 out]
          }
          frame True {
            w589 = u16 10 items=["1.0"=10, "1.5"=15, "2.0"=20] ("stop bits (10: 1 bit)")
            n258 = Decrement(x=w585) -> (x-1=w584:i32)
            n259 = Multiply(x=w584, y=5) -> (x*y=w572:i32)
            n260 = for {
              N: 3 -> [_]
              tunnel: w572 -> [w596]
              i -> [w595]
              n261 = Add(x=w596, y=w595) -> (x+y=w597:i32)
              n262 = Increment(x=w597) -> (x+1=w606:i32)
              n263 = Quotient & Remainder(x=w606, y=u16 5) -> (x-y*floor(x/y)=w602:i32, floor(x/y)=w603:i32)
              n264 = Greater Than 0?(x=w602) -> (x > 0?=w604:bool)
              n265 = case shown="真" w604 {
                tunnel: w603 -> [w608 w617]
                tunnel: w602 -> [_ w615]
                tunnel: [w607 w611] -> w600
                frame False {
                  n266 = Number To Decimal String(number=w608) -> (decimal integer string=w610:string)  [unwired: 1 in]
                  n267 = Concatenate Strings(w610, "-5" ("字符串")) -> (w607:string)
                }
                frame True {
                  n268 = Increment(x=w617) -> (x+1=w616:i32)
                  n269 = Number To Decimal String(number=w615) -> (decimal integer string=w612:string)  [unwired: 1 in]
                  n270 = Number To Decimal String(number=w616) -> (decimal integer string=w614:string)  [unwired: 1 in]
                  n271 = Concatenate Strings(w614, "-" ("字符串"), w612) -> (w611:string)
                }
              }
              n272 = control-ref of="本VI"() -> (w601:refnum<vi>)
              n273 = To Variant(anything=TRUE) -> (Variant=w598:variant)
              n274 = invoke class="VI" method="Ctrl Val.Set"(reference=w601, "Control Name"=w600, "Value"=w598) -> ()  [unwired: 2 in, 5 out]
            }
            n275 = property on="控制板" class="VISAName"() -> ("Value"=w588:refnum<visa-resource-name>)  [unwired: 2 in, 2 out]
            n276 = call-poly "VISA Configure Serial Port"("VISA resource name"=w588, "baud rate (9600)"=u32 38400, "data bits (8)"=u16 8, "parity (0:none)"=enum16{"None", "Odd", "Even", "Mark", "Space"}."None", "stop bits (10: 1 bit)"=w589) -> ("VISA resource name out"=w593:refnum<visa-resource-name>)  [unwired: 9 in, 1 out]
            n277 = Add(x=w572, y=0) -> (x+y=w574:i32)
            n278 = VISA Open(VISA resource name=w593) -> (VISA resource name=w587:refnum<visa-resource-name>)  [unwired: 4 in, 1 out]
            n279 = flat-sequence {
              tunnel: [w620] -> w594
              tunnel: w574 -> [w619]
              tunnel: w587 -> [w618]
              tunnel: w594 -> [w621]
              tunnel: [w621] -> w586
              tunnel: w586 -> [w625]
              tunnel: [w624] -> w579
              tunnel: w577 -> [w623]
              tunnel: w579 -> [w626]
              tunnel: [w626] -> w578
              tunnel: w580 -> [w630]
              tunnel: w578 -> [w629]
              tunnel: [w628] -> w576
              frame #0 {
                n280 = call "controll_single.vi"("控制编号"=w619, "VISA资源名称"=w618) -> ("VISA资源名称输出"=w620:refnum<visa-resource-name>)  [unwired: 9 in]
              }
              frame #1 {
                n281 = Wait (ms)(milliseconds to wait=u32 50 ("等待时间（毫秒）")) -> ()  [unwired: 1 out]
              }
              frame #2 {
                n282 = call "controll_single.vi"("控制编号"=w623, "VISA资源名称"=w625) -> ("VISA资源名称输出"=w624:refnum<visa-resource-name>)  [unwired: 9 in]
              }
              frame #3 {
                n283 = Wait (ms)(milliseconds to wait=u32 50 ("等待时间（毫秒）")) -> ()  [unwired: 1 out]
              }
              frame #4 {
                n284 = call "controll_single.vi"("控制编号"=w630, "VISA资源名称"=w629) -> ("VISA资源名称输出"=w628:refnum<visa-resource-name>)  [unwired: 9 in]
              }
              frame #5 {
                n285 = Wait (ms)(milliseconds to wait=u32 50 ("等待时间（毫秒）")) -> ()  [unwired: 1 out]
              }
            }
            n286 = Add(x=w572, y=1) -> (x+y=w577:i32)
            n287 = Add(x=w572, y=2) -> (x+y=w580:i32)
            n288 = VISA Close(VISA resource name=w576) -> ()  [unwired: 1 in, 1 out]
          }
        }
      }
      event "退出": Value Change {
        n289 = event-data() -> ("NewVal"=w632:bool)  [unwired: 1 in, 5 out]
        n290 = case shown="真" w632 {
          frame False {
          }
          frame True {
            n291 = flat-sequence {
              tunnel: [w637] -> w634
              frame #0 {
                n292 = property on="控制板" class="VISAName"() -> ("Value"=w635:refnum<visa-resource-name>)  [unwired: 2 in, 2 out]
                n293 = VISA Close(VISA resource name=w635) -> ()  [unwired: 1 in, 1 out]
                n294 = property on="退出" class="Bool (严格)"("Value"=FALSE ("退出")) -> ()  [unwired: 2 in, 2 out]
              }
              frame #1 {
                n295 = control-ref of="本VI"() -> (w637:refnum<vi>)
              }
            }
            n296 = invoke class="VI" method="FP.Close"(reference=w634) -> (reference out=w633:refnum<vi>)  [unwired: 2 in, 2 out]
            n297 = invoke class="VI" method="Abort VI"(reference=w633) -> ()  [unwired: 2 in, 3 out]
          }
        }
      }
    }
  }
  n298 = property on="开" class="Ring (严格)"("Strings []"=w1) -> ()  [unwired: 2 in, 2 out]
  n299 = property on="关" class="Ring (严格)"("Strings []"=w1) -> ()  [unwired: 2 in, 2 out]
